vi "Template Path.vi"(9 "Template Name":string, 10 "Base Path":path) -> (2 "Template Path":path)   [LabVIEW 2021, in "_Create From Template.lvlib"]
uses:
  _Create From Template.lvlib
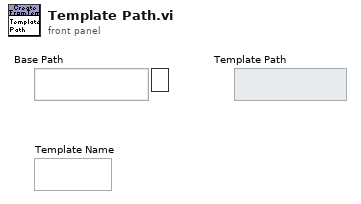
[diagram p1: front panel]
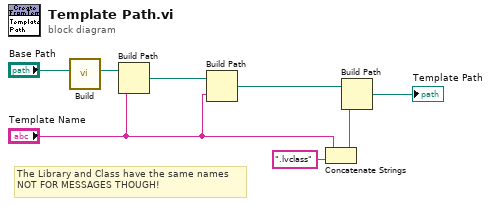
[diagram p0: block diagram]
diagram:
  # "The Library and Class have the same names\nNOT FOR MESSAGES THOUGH!"
  n1 = call "Build.vi"("Base Path"="Base Path") -> ("Templates Path"=w4:path)  [unwired: 10 in]
  n2 = Build Path(base path=w4, name or relative path="Template Name") -> (appended path=w3:path)
  n3 = Build Path(base path=w3, name or relative path="Template Name") -> (appended path=w2:path)
  n4 = Concatenate Strings("Template Name", ".lvclass" ("string")) -> (w6:string)
  n5 = Build Path(base path=w2, name or relative path=w6) -> (appended path=→"Template Path":path)
